vi "Calculate Shoot Speed.vi"(9 "Manual Override":bool, 10 "Driver Shoot":bool, 11 "Joystick":T1) -> ()   [LabVIEW 2011]
uses:
  Team Code/Robot Global Data.vi
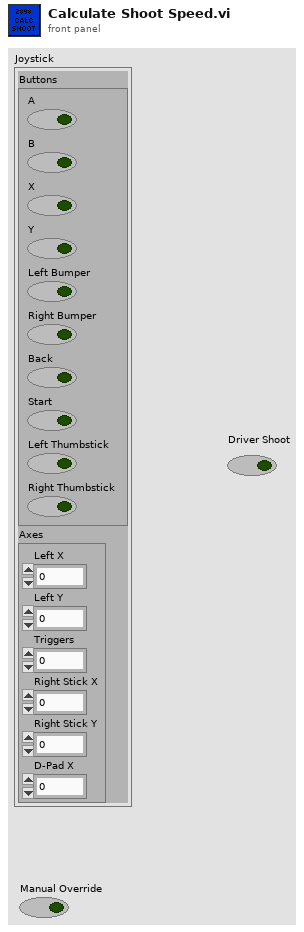
[diagram p1: front panel]
types:
  T1 = cluster{"Buttons":cluster{"A":bool, "B":bool, "X":bool, "Y":bool, "Left Bumper":bool, "Right Bumper":bool, "Back":bool, "Start":bool, "Left Thumbstick":bool, "Right Thumbstick":bool}, "Axes":cluster{"Left X ":dbl, "Left Y":dbl, "Triggers":dbl, "Right Stick X":dbl, "Right Stick Y":dbl, "D-Pad X":dbl}}
  T2 = enum16{"Camera Shot", "Manual Override Shot", "Full Speed Shot", "Key Shot", "Fender Shot", "Stop"}
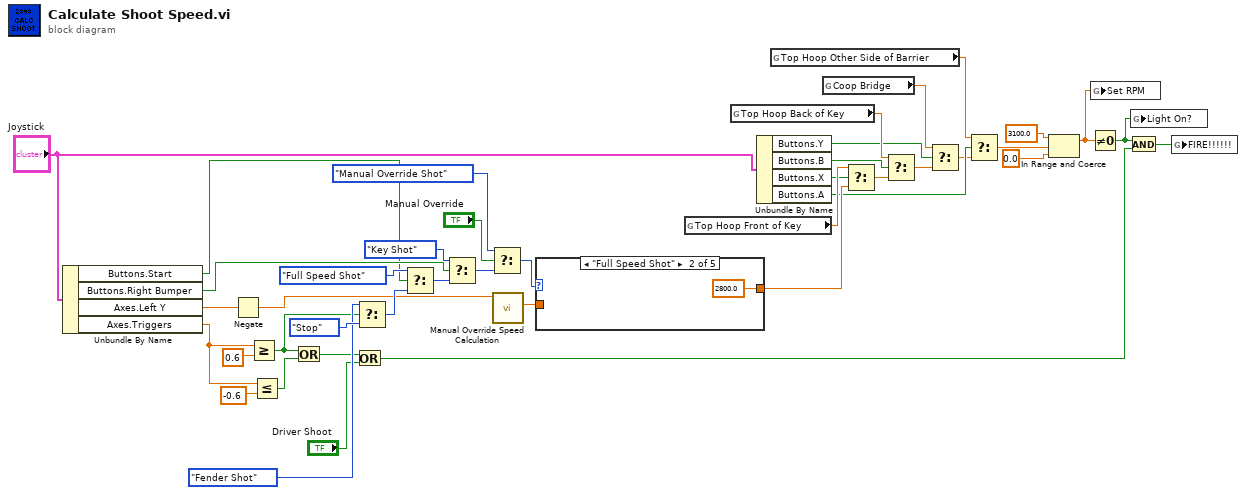
[diagram p0: block diagram]
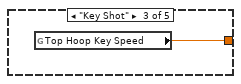
[diagram p3: hidden frame]
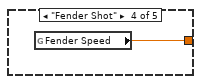
[diagram p4: hidden frame]
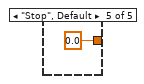
[diagram p5: hidden frame]
diagram:
  n1 = Unbundle By Name("Joystick") -> ("Buttons.Start"=w28:bool, "Buttons.Right Bumper"=w29:bool, "Axes.Left Y"=w42:dbl, "Axes.Triggers"=w23:dbl)
  n2 = Negate(x=w42) -> (-x=w17:dbl)
  n3 = Greater Or Equal?(x=w23, y=0.6) -> (x >= y?=w21:bool)
  n4 = Less Or Equal?(x=w23, y=-0.6) -> (x <= y?=w24:bool)
  n5 = Or(x=w21, y=w24) -> (x .or. y?=w19:bool)
  n6 = Or(x=w19, y="Driver Shoot") -> (x .or. y?=w18:bool)
  n7 = Select(t=T2."Fender Shot" ("Shooting Mode"), s=w21, f=T2."Stop" ("Shooting Mode")) -> (s? t:f=w32:T2)
  n8 = Select(t=T2."Full Speed Shot" ("Shooting Mode"), s=w28, f=w32) -> (s? t:f=w30:T2)
  n9 = Select(t=T2."Key Shot" ("Shooting Mode"), s=w29, f=w30) -> (s? t:f=w39:T2)
  n10 = Select(t=T2."Manual Override Shot" ("Shooting Mode"), s="Manual Override", f=w39) -> (s? t:f=w38:T2)
  n11 = call "Manual Override Speed Calculation.vi"("Input"=w17) -> ("Output"=w16:dbl)  [unwired: 10 in]
  n12 = case shown="\"Full Speed Shot\"" w38 {
    tunnel: [w43 2800.0 ("Fender Speed") w45 w46 0.0] -> w10
    tunnel: w16 -> [w43 _ _ _ _]
    frame "Manual Override Shot" {
    }
    frame "Full Speed Shot" {
    }
    frame "Key Shot" {
      n13 = global read "Robot Global Data.vi" "Top Hoop Key Speed"() -> (w45:dbl)
    }
    frame "Fender Shot" {
      n14 = global read "Robot Global Data.vi" "Fender Speed"() -> (w46:dbl)
    }
    frame "Stop", Default {
    }
  }
  n15 = global read "Robot Global Data.vi" "Top Hoop Front of Key"() -> (w11:dbl)
  n16 = global read "Robot Global Data.vi" "Top Hoop Back of Key"() -> (w12:dbl)
  n17 = Unbundle By Name("Joystick") -> ("Buttons.Y"=w8:bool, "Buttons.B"=w6:bool, "Buttons.X"=w7:bool, "Buttons.A"=w4:bool)
  n18 = global read "Robot Global Data.vi" "Top Hoop Other Side of Barrier"() -> (w1:dbl)
  n19 = global read "Robot Global Data.vi" "Coop Bridge"() -> (w13:dbl)
  n20 = Select(t=w11, s=w7, f=w10) -> (s? t:f=w14:dbl)
  n21 = Select(t=w12, s=w6, f=w14) -> (s? t:f=w15:dbl)
  n22 = Select(t=w13, s=w8, f=w15) -> (s? t:f=w3:dbl)
  n23 = Select(t=w1, s=w4, f=w3) -> (s? t:f=w2:dbl)
  n24 = In Range and Coerce(upper limit=3100.0, x=w2, lower limit=0.0) -> (coerced(x)=w27:dbl)  [unwired: 1 out]
  n25 = Not Equal To 0?(x=w27) -> (x != 0?=w5:bool)
  n26 = global write "Robot Global Data.vi" "Set RPM"(w27) -> ()
  n27 = And(x=w5, y=w18) -> (x .and. y?=w25:bool)
  n28 = global write "Robot Global Data.vi" "Light On?"(w5) -> ()
  n29 = global write "Robot Global Data.vi" "FIRE!!!!!!"(w25) -> ()
